vi "Ramp to Set.vi"(6 "Axis":T1, 8 "error in (no error)":errorcluster, 11 "Instrument.VRM in":refnum<class "Instrument.OxfordVRM.lvclass">) -> (0 "error out":errorcluster, 2 "Response":string, 3 "Instrument.VRM out":refnum<class "Instrument.OxfordVRM.lvclass">)   [LabVIEW 2019, in "Instrument.OxfordVRM.lvclass"]
uses:
  Instrument.OxfordVRM.lvclass
  Typedefs/VRM Magnet Axis--Enum.ctl
  <instrlib>/Mercury iXX/Public/Libraries/Magnet/Controls/PSU Actions.ctl
  Typedefs/Instrument.VRM.Commands-enum.ctl
  Typedefs/VRM Action-Axis--Cluster.ctl
  74560bd0-e206-4b39-9b04-00724d861558.vi
  74560bd0-e206-4b39-9b04-00724d861558.vi/b0d3ef14-0649-4982-b2d0-3ff109e814f4.vi
  74560bd0-e206-4b39-9b04-00724d861558.vi/b0d3ef14-0649-4982-b2d0-3ff109e814f4.vi/7a1fe5f9-6bae-4c38-8687-93b226639de0.vi
  74560bd0-e206-4b39-9b04-00724d861558.vi/b0d3ef14-0649-4982-b2d0-3ff109e814f4.vi/0dcc6473-5b22-4f0b-b170-3fb6b215bfd1.vi
  74560bd0-e206-4b39-9b04-00724d861558.vi/b0d3ef14-0649-4982-b2d0-3ff109e814f4.vi/0dcc6473-5b22-4f0b-b170-3fb6b215bfd1.vi/a8c26276-2d1d-49a3-9eb1-d1e552ccdbee.vi
  74560bd0-e206-4b39-9b04-00724d861558.vi/b0d3ef14-0649-4982-b2d0-3ff109e814f4.vi/0dcc6473-5b22-4f0b-b170-3fb6b215bfd1.vi/f8b30c0b-7ccb-4db2-8e8c-d0ed993a0804.vi
  <userlib>/LevyLab/Levylab Instruments/SMOs/RemoteControl/API/Remote Client.vi
  <vilib>/JDP Science/JSONtext/JSON text to Variant.vi
  <vilib>/JDP Science/JSONtext/LVClass Serializer/JSONtext LVClass Serializer.lvclass
  <instrlib>/Mercury iXX/Public/Libraries/Magnet.lvlib
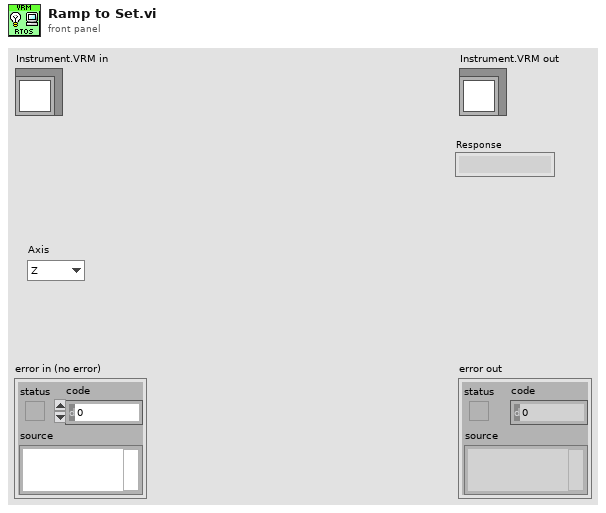
[diagram p1: front panel]
types:
  T1 = typedef "Instrument.OxfordVRM.lvclass/VRM Magnet Axis--Enum.ctl" = enum16{"Z", "X", "Y", "ALL"}
  T2 = typedef "Instrument.OxfordVRM.lvclass/VRM Action-Axis--Cluster.ctl" = cluster{"PSU Act Stat":T3, "Axis":T1}
  T3 = typedef "Mercury iXX.lvlib/Magnet.lvlib/PSU Actions.ctl" = string
  T4 = typedef "Instrument.OxfordVRM.lvclass/Instrument.VRM.Commands-enum.ctl" = enum16{"setAction", "setTarget", "setMagnetField", "getStatus", "getTarget", "getMagnetField"}
  T5 = cluster{"Holding":bool, "Ramp to Setpoint":bool, "Ramp to Zero":bool, "Clamp":bool}
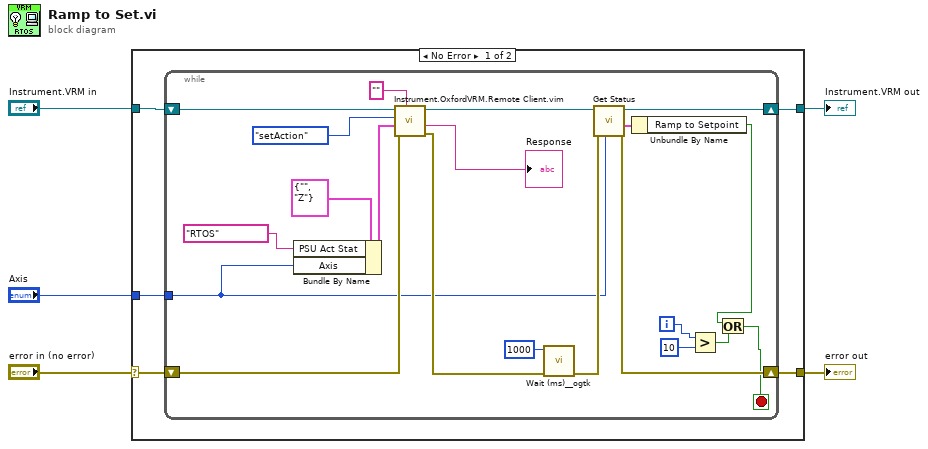
[diagram p0: block diagram]
diagram:
  n1 = case shown="No Error" "error in (no error)" {
    selector: "error in (no error)" -> [w9 w33]
    tunnel: [w8 w33] -> w4
    tunnel: [w7 w32] -> w2
    tunnel: "Instrument.VRM in" -> [w10 w32]
    tunnel: "Axis" -> [w6 _]
    frame No Error {
      n2 = while {
        shift-right: [w26] -> w7
        shift-left: w10 -> [w25]
        shift-right: [w27] -> w8
        shift-left: w9 -> [w31]
        tunnel: w6 -> [w15]
        i -> [w13]
        stop <- w21 stop-if-true
        n3 = Bundle By Name(cluster=T2 {"PSU Act Stat"="", "Axis"=enum."Z"} ("Action"), "PSU Act Stat"=T3 "RTOS", "Axis"=w15) -> (w14:T2)
        n4 = call "Instrument.OxfordVRM.Remote Client.vim"("Data Out type"="", "error in (no error)"=w31, "Data"=w14, "Commands"=Instrument.VRM.Commands-enum."setAction", "Instrument.VRM in"=w25) -> ("error out"=w20:errorcluster, "Data out"=→"Response":string, "Instrument.VRM out"=w19:refnum<class "Instrument.OxfordVRM.lvclass">)  [unwired: 4 in]
        n5 = call <userlib>:"Wait (ms)__ogtk.vi"("error in (no error)"=w20, "milliseconds to wait"=u32 1000) -> ("error out"=w28:errorcluster)  [unwired: 8 in, 1 out]
        n6 = call "Get Status.vi"("Axis"=w15, "error in (no error)"=w28, "Instrument.VRM in"=w19) -> ("error out"=w27:errorcluster, "Status (ALL)"=w29:T5, "Instrument.VRM out"=w26:refnum<class "Instrument.OxfordVRM.lvclass">)  [unwired: 5 in, 1 out]
        n7 = Unbundle By Name(w29) -> ("Ramp to Setpoint"=w22:bool)
        n8 = Greater?(x=w13, y=10) -> (0:w23:bool)
        n9 = Or(x=w22, y=w23) -> (x .or. y?=w21:bool)
      }
    }
    frame Error {
    }
  }
  "error out" <- w4
  "Instrument.VRM out" <- w2
